vi "升降桅杆.vi"() -> ()   [LabVIEW 2018]
panel:
  in  "停止 2":bool
  in  "抱紧 2":bool
  in  "打开 2":bool
  in  "停止":bool
  in  "抱紧":bool
  in  "打开":bool
  out "推进模块故障 2":bool caption="地位正常运行"
  out "推进模块正常 2":bool
  in  "停止":bool
  in  "选项卡控件 8":T1(tab)
  out "回转故障信息":string
  in  "停止 3":bool
  in  "原始位":bool
  in  "工作位":bool
  out "到达工作位":bool
  out "电机运行状态 4":bool
  out "未到位 4":bool
  out "到达原始位":bool
  out "回转模块故障":bool caption="地位正常运行"
  out "回转模块正常":bool
  out "俯仰位移传感器":i64 caption="Output Value"
  out "挡板推进传感器":i64 caption="Output Value"
  out "升降桅杆位移传感器":i64 caption="Output Value"
  out "推进模块故障信息":string
  out "电机运行状态 3":bool
  out "未到位 3":bool
  out "缩回到位":bool
  out "推进到位":bool
  out "Output Value 18":dbl caption="Output Value" format="%.2f"
  out "Output Value 17":dbl caption="Output Value" format="%.2f"
  out "Output Value 16":dbl caption="Output Value" format="%.2f"
  out "Output Value 15":dbl caption="Output Value" format="%.2f"
  out "Output Value 14":dbl caption="Output Value" format="%.2f"
  out "Output Value 13":dbl caption="Output Value" format="%.2f"
  out "Output Value 12":dbl caption="Output Value" format="%.2f"
  out "Output Value 11":dbl caption="Output Value" format="%.2f"
  out "Output Value 10":dbl caption="Output Value" format="%.2f"
  out "Output Value 9":dbl caption="Output Value" format="%.2f"
  out "Output Value 8":dbl caption="Output Value" format="%.2f"
  out "Output Value 7":dbl caption="Output Value" format="%.2f"
  out "Output Value 6":dbl caption="Output Value" format="%.2f"
  out "Output Value 5":dbl caption="Output Value" format="%.2f"
  out "Output Value 4":dbl caption="Output Value" format="%.2f"
  out "Output Value 3":dbl caption="Output Value" format="%.2f"
  out "Output Value 2":dbl caption="Output Value" format="%.2f"
  out "Output Value":dbl format="%.2f"
  out "系统通讯故障":bool
  out "系统通讯正常":bool
  in  "灯56":bool
  in  "灯34":bool
  in  "灯12":bool
  out "电机运行状态 2":bool
  out "未到位 2":bool
  out "抱爪抱紧到位 2":bool
  out "抱爪打开到位 2":bool
  out "电机运行状态":bool
  out "未到位":bool
  out "抱爪抱紧到位":bool
  out "抱爪打开到位":bool
  out "电机或驱动器故障 2":bool
  out "电机或驱动器正常 2":bool
  out "电机或驱动器故障":bool
  out "电机或驱动器正常":bool
  out "挡板后退到位":bool
  out "挡板推进到位":bool
  out "俯仰缸回降到位":bool
  out "俯仰缸升起到位":bool
  out "桅杆位置4到位":bool
  out "桅杆位置3到位":bool
  out "桅杆位置2到位":bool
  out "桅杆位置1到位":bool
  in  "挡板后退":bool
  in  "挡板推进":bool
  in  "俯仰缸回降":bool
  in  "俯仰缸升起":bool
  in  "桅杆位置":bool
  in  "桅杆位置3":bool
  in  "桅杆位置2":bool
  in  "桅杆位置1":bool
  in  "Application filename":string="canceshi1"
  in  "IP Port":string="22222"
  in  "IP Address":string="192.168.0.10"
  out "旋转":dbl caption="Output Value" format="%.2f"
  out "升降":dbl caption="Output Value" format="%.2f"
  out "抱爪1":dbl caption="Output Value" format="%.2f"
  out "伺服阀":dbl caption="Output Value" format="%.2f"
  out "startapp":i32 caption="port copy"
  out "loadapp":i32 caption="port copy"
  out "tcpip":i32 caption="Port"
  # "推进控制模块"
  # "回转控制模块"
  # "捕获臂控制模块"
  # "单位/mm"
  # "单位/mm"
  # "单位/mm"
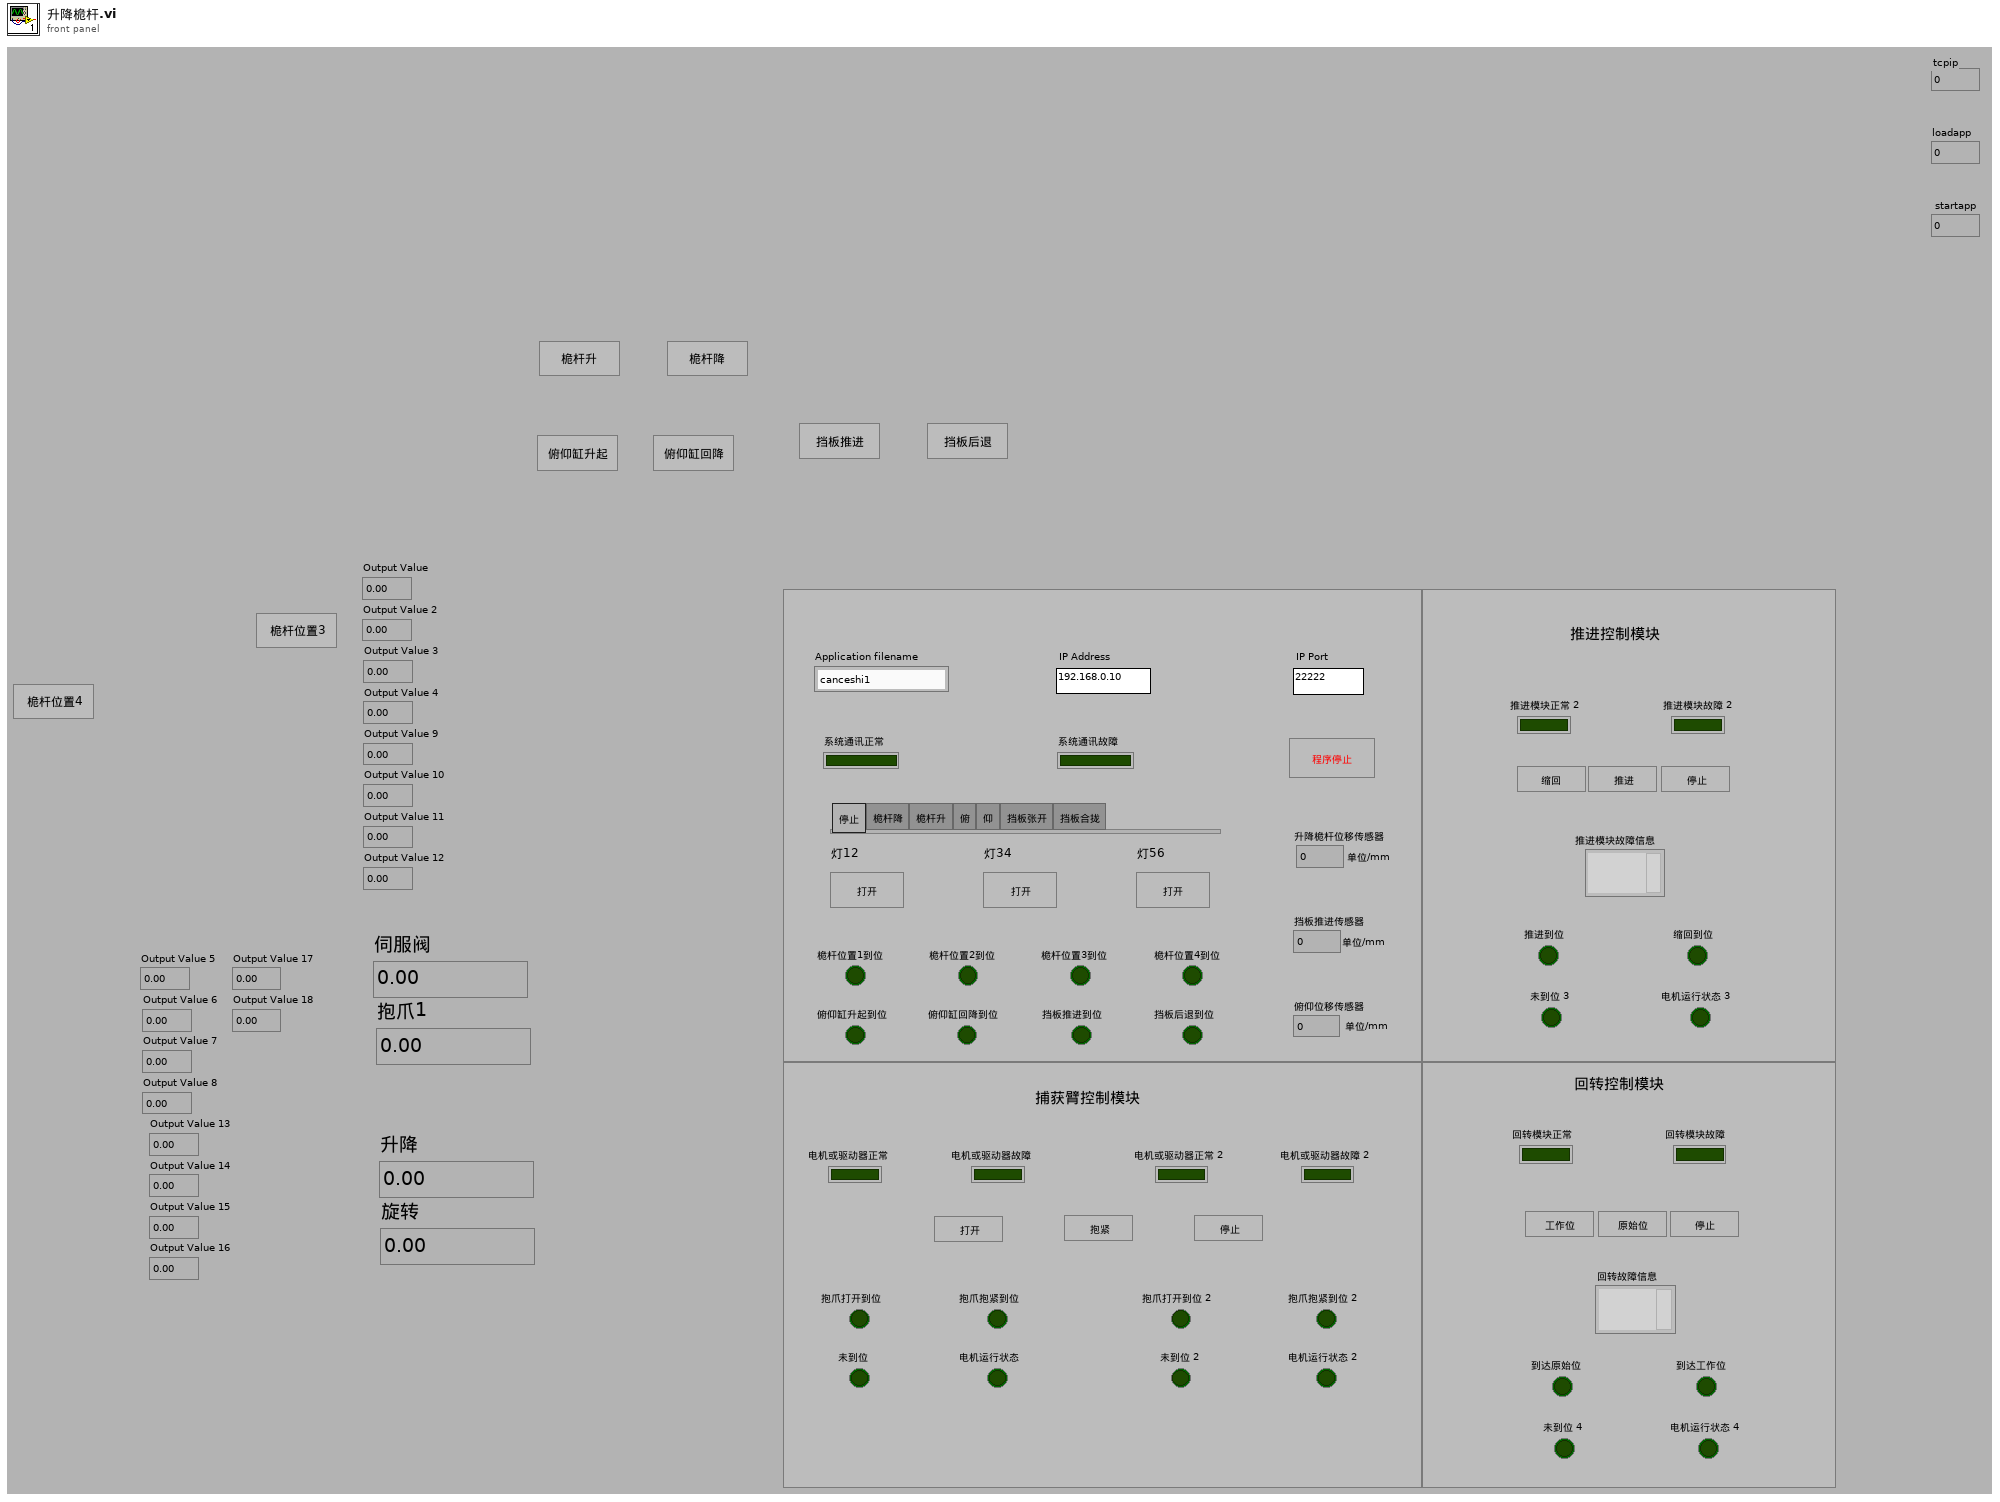
[diagram p1: front panel]
types:
  T1 = enum32{"停止", "桅杆降", "桅杆升", "俯", "仰", "挡板张开", "挡板合拢"}
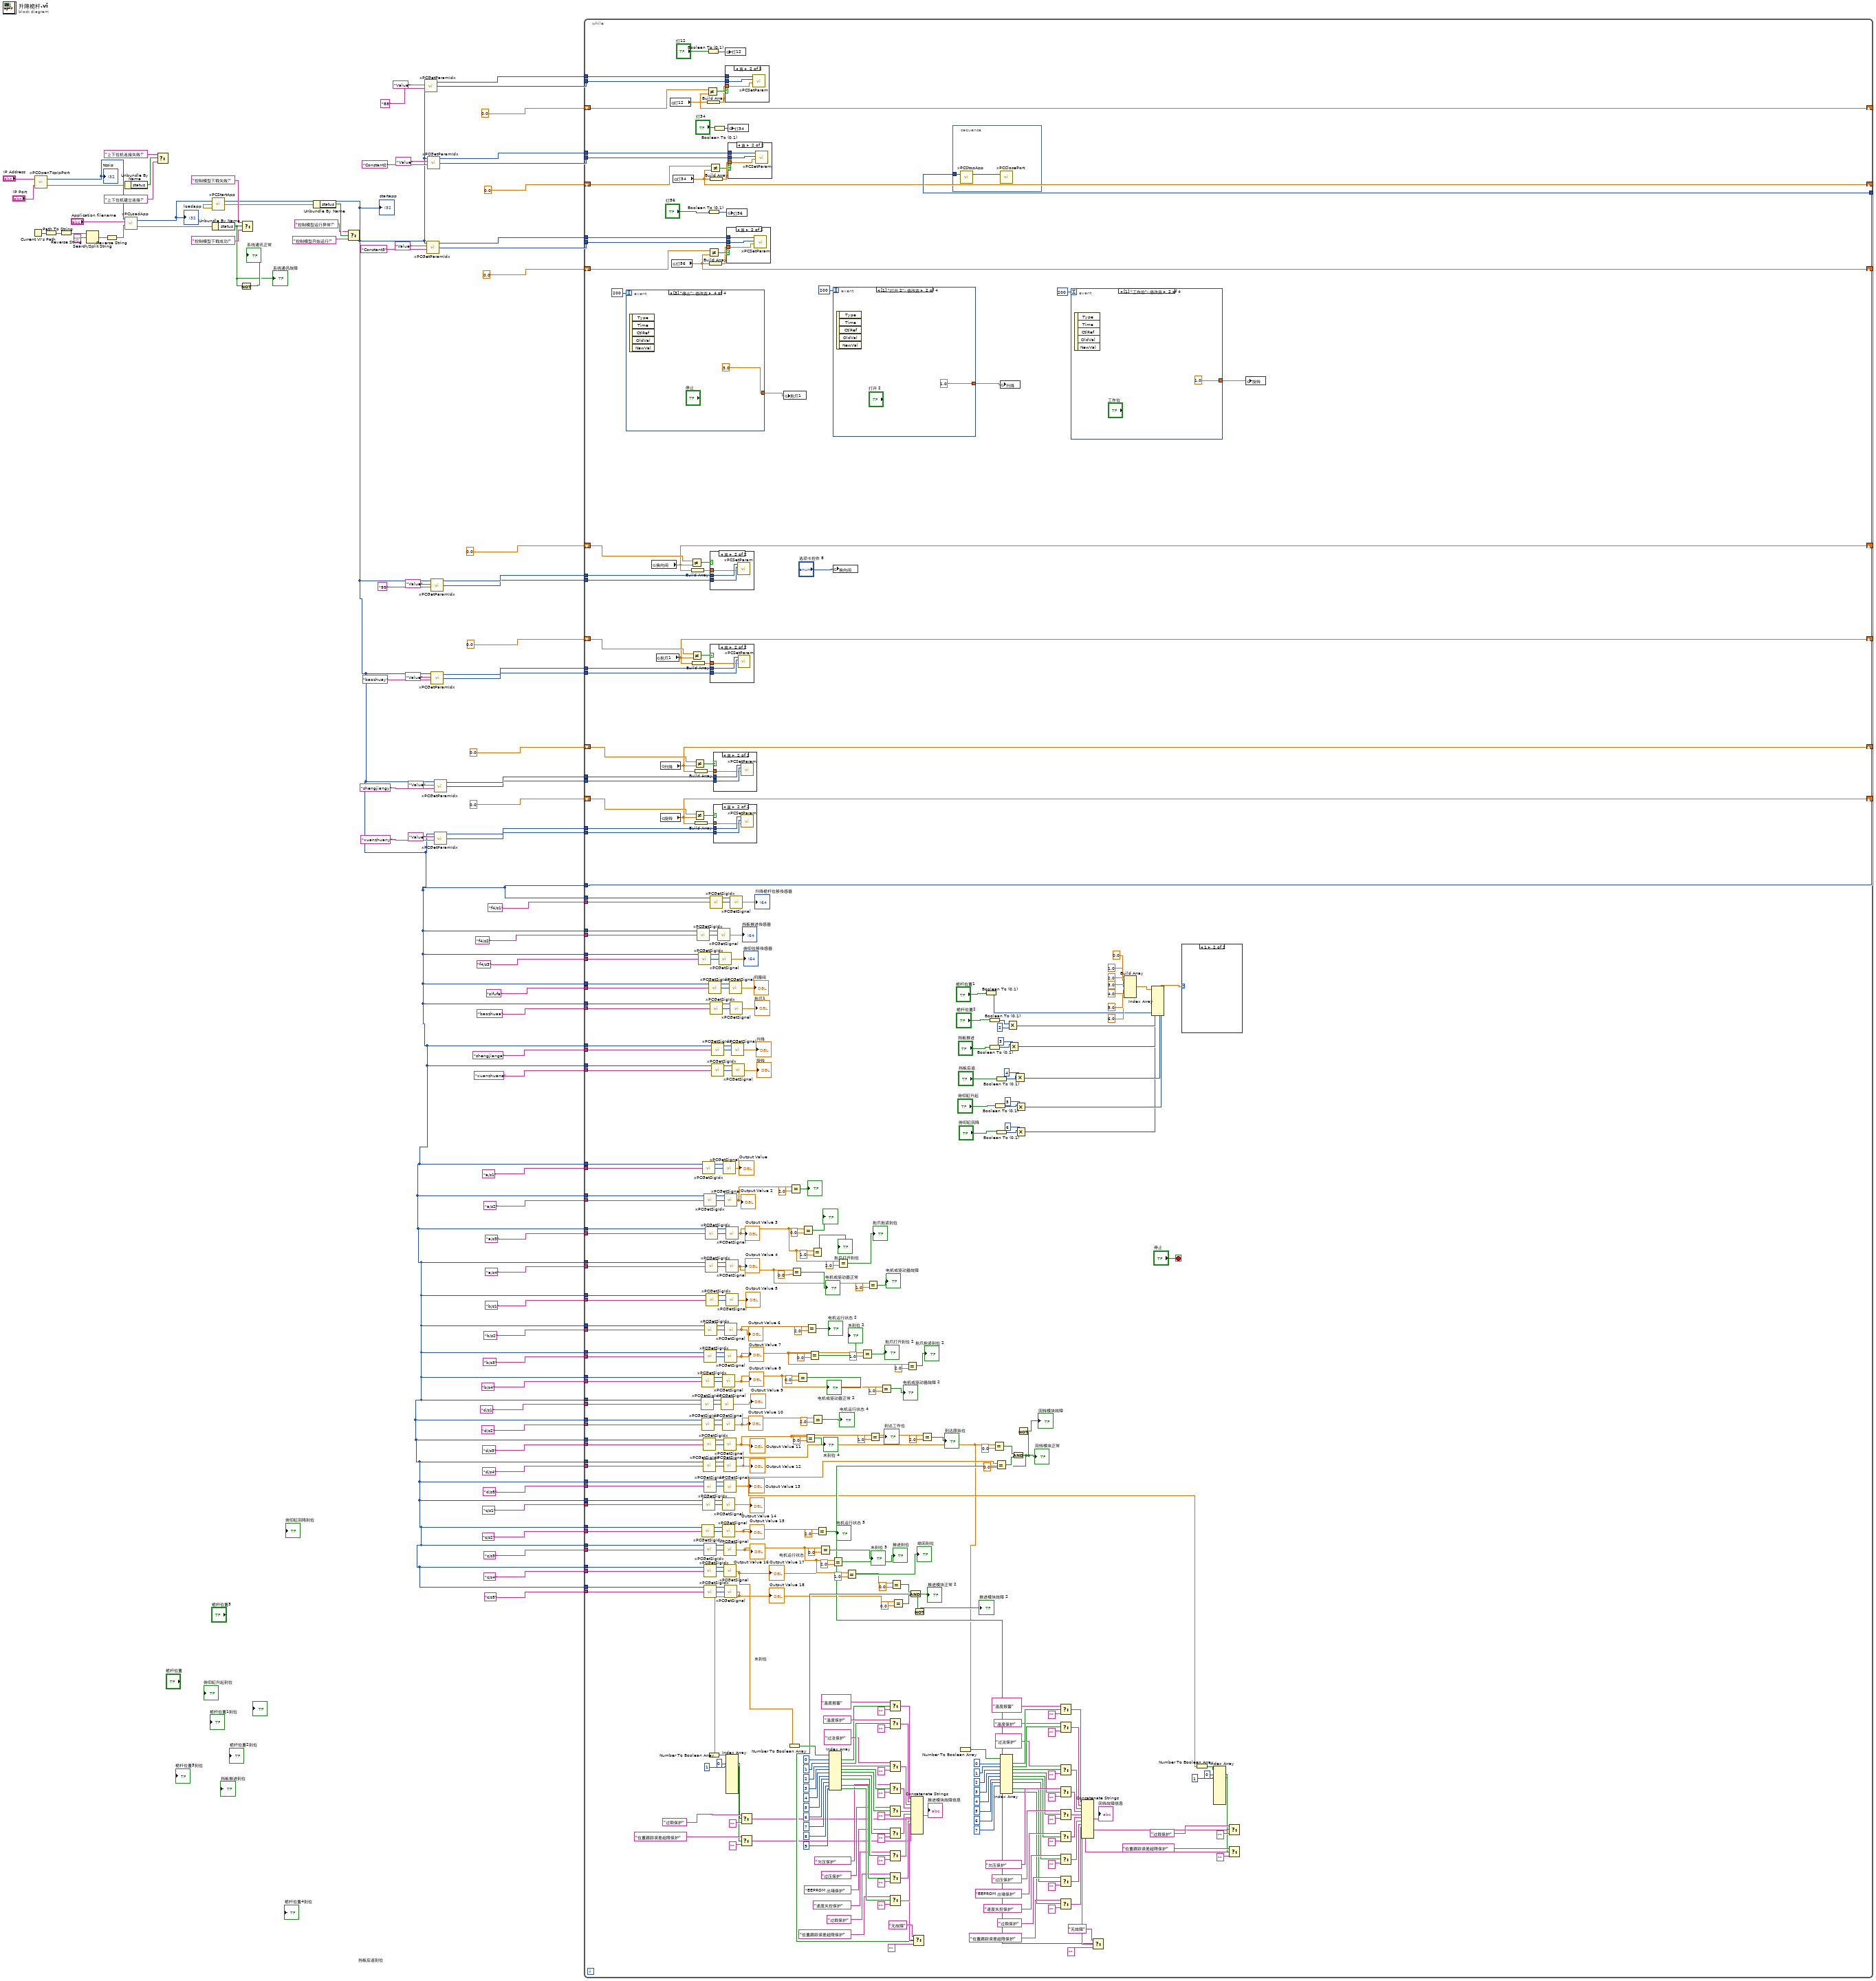
[diagram p0: block diagram]
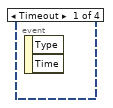
[diagram p2: hidden frame]
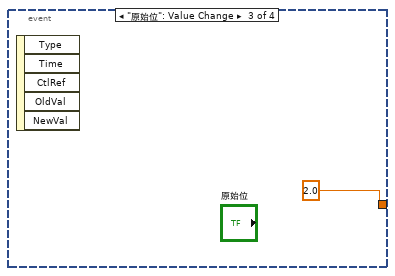
[diagram p3: hidden frame]
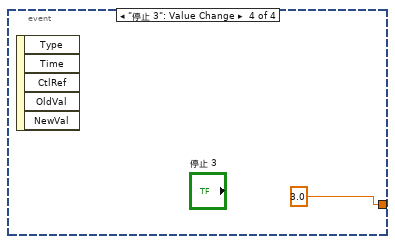
[diagram p4: hidden frame]
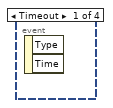
[diagram p5: hidden frame]
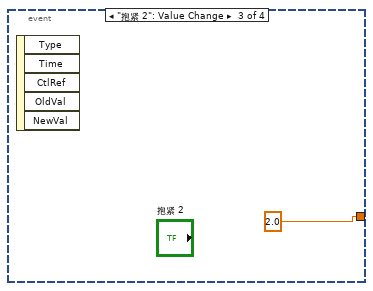
[diagram p6: hidden frame]
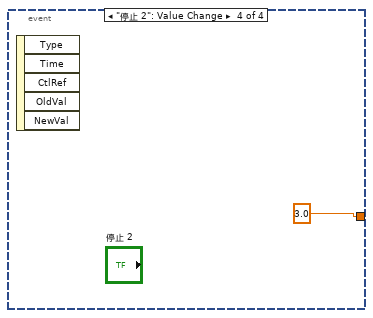
[diagram p7: hidden frame]
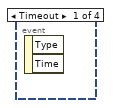
[diagram p8: hidden frame]
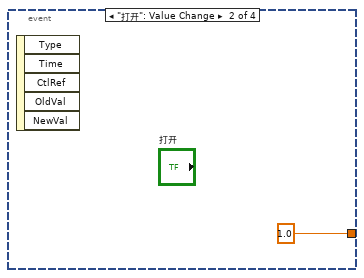
[diagram p9: hidden frame]
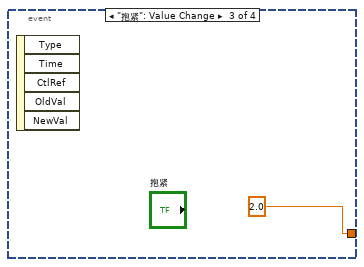
[diagram p10: hidden frame]
diagram:
  n1 = Current VI's Path() -> (path=w80:path)
  n2 = call "xPCOpenTcpIpPort.vi"("port"="IP Port", "address"="IP Address") -> ("error out"=w70:errorcluster, "Port"=w71:i32)
  "tcpip" <- w71
  n3 = Path To String(path=w80) -> (string=w82:string)
  n4 = Reverse String(1:w82) -> (0:w84:string)
  n5 = Search/Split String(string=w84, search string/char (-)="\\" ("search char (-)")) -> (match + rest of string=w83:string)  [unwired: 1 in, 2 out]
  n6 = Reverse String(1:w83) -> (0:w85:string)
  n7 = Unbundle By Name(w70) -> ("status"=w77:bool)
  n8 = call "xPCLoadApp.vi"("pathstr"=w85, "filename"="Application filename", "port"=w71) -> ("error out"=w72:errorcluster, "port copy"=w79:i32)  [unwired: 1 in]
  "loadapp" <- w79
  n9 = Select(t="上下位机连接失败!" ("message"), s=w77, f="上下位机建立连接!" ("message")) -> ()  [unwired: 1 out]
  n10 = call "xPCStartApp.vi"("port"=w79) -> ("error out"=w64:errorcluster, "port copy"=w1:i32)  [unwired: 1 in]
  "startapp" <- w1
  n11 = Unbundle By Name(w72) -> ("status"=w37:bool)
  "系统通讯故障" <- w37
  n12 = Not(x=w37) -> (.not. x?=→"系统通讯正常":bool)
  n13 = Select(t="控制模型下载失败!" ("message"), s=w37, f="控制模型下载成功!" ("message")) -> ()  [unwired: 1 out]
  n14 = Unbundle By Name(w64) -> ("status"=w66:bool)
  n15 = Select(t="控制模型运行异常!" ("message"), s=w66, f="控制模型开始运行!" ("message")) -> ()  [unwired: 1 out]
  n16 = call "xPCGetParamIdx.vi"("blockpath"="88" ("pathstr"), "parametername"="Value" ("filename"), "port"=w1) -> ("identifier"=w57:i32, "port copy"=w58:i32)  [unwired: 1 in, 1 out]
  n17 = call "xPCGetParamIdx.vi"("blockpath"="Constant3" ("pathstr"), "parametername"="Value" ("filename"), "port"=w1) -> ("identifier"=w46:i32, "port copy"=w47:i32)  [unwired: 1 in, 1 out]
  n18 = call "xPCGetParamIdx.vi"("blockpath"="Constant2" ("pathstr"), "parametername"="Value" ("filename"), "port"=w1) -> ("identifier"=w51:i32, "port copy"=w50:i32)  [unwired: 1 in, 1 out]
  n19 = call "xPCGetParamIdx.vi"("blockpath"="99" ("pathstr"), "parametername"="Value" ("filename"), "port"=w1) -> ("identifier"=w43:i32, "port copy"=w61:i32)  [unwired: 1 in, 1 out]
  n20 = call "xPCGetParamIdx.vi"("blockpath"="baozhuay" ("pathstr"), "parametername"="Value" ("filename"), "port"=w1) -> ("identifier"=w16:i32, "port copy"=w14:i32)  [unwired: 1 in, 1 out]
  n21 = call "xPCGetParamIdx.vi"("blockpath"="shengjiangy" ("pathstr"), "parametername"="Value" ("filename"), "port"=w1) -> ("identifier"=w7:i32, "port copy"=w9:i32)  [unwired: 1 in, 1 out]
  n22 = call "xPCGetParamIdx.vi"("blockpath"="xuanzhuany" ("pathstr"), "parametername"="Value" ("filename"), "port"=w1) -> ("identifier"=w6:i32, "port copy"=w4:i32)  [unwired: 1 in, 1 out]
  n23 = while {
    tunnel: w1 -> [w473]
    tunnel: [w473] -> w78
    shift-right: [w467] -> _
    shift-left: 0.0 -> [w470]
    tunnel: w43 -> [w469]
    tunnel: w61 -> [w468]
    shift-right: [w466] -> _
    shift-left: 0.0 -> [w465]
    tunnel: w57 -> [w462]
    tunnel: w58 -> [w461]
    tunnel: w1 -> [w458]
    tunnel: "f4/s1" ("pathstr") -> [w455]
    shift-right: [w448] -> _
    shift-left: 0.0 -> [w449]
    tunnel: w51 -> [w452]
    tunnel: w50 -> [w453]
    shift-right: [w447] -> _
    shift-left: 0.0 -> [w446]
    tunnel: w46 -> [w443]
    tunnel: w47 -> [w442]
    tunnel: w1 -> [w433]
    tunnel: "sifufa" ("pathstr") -> [w436]
    tunnel: w1 -> [w432]
    tunnel: "baozhuaa" ("pathstr") -> [w429]
    tunnel: w1 -> [w427]
    tunnel: "shengjianga" ("pathstr") -> [w424]
    tunnel: w1 -> [w418]
    tunnel: "xuanzhuana" ("pathstr") -> [w421]
    tunnel: w1 -> [w393]
    tunnel: "a/s1" ("pathstr") -> [w391]
    tunnel: w1 -> [w394]
    tunnel: "a/s2" ("pathstr") -> [w396]
    tunnel: w1 -> [w401]
    tunnel: "a/s3" ("pathstr") -> [w399]
    tunnel: w1 -> [w402]
    tunnel: "a/s4" ("pathstr") -> [w404]
    tunnel: w1 -> [w409]
    tunnel: "b/s1" ("pathstr") -> [w407]
    tunnel: w1 -> [w410]
    tunnel: "b/s2" ("pathstr") -> [w412]
    tunnel: w1 -> [w417]
    tunnel: "b/s3" ("pathstr") -> [w415]
    tunnel: w1 -> [w389]
    tunnel: "b/s4" ("pathstr") -> [w387]
    tunnel: w1 -> [w382]
    tunnel: "d/s1" ("pathstr") -> [w384]
    tunnel: w1 -> [w381]
    tunnel: "d/s2" ("pathstr") -> [w379]
    tunnel: w1 -> [w374]
    tunnel: "d/s3" ("pathstr") -> [w376]
    tunnel: w1 -> [w373]
    tunnel: "d/s4" ("pathstr") -> [w371]
    tunnel: w1 -> [w366]
    tunnel: "d/s5" ("pathstr") -> [w368]
    tunnel: w1 -> [w365]
    tunnel: "c/s1" ("pathstr") -> [w363]
    tunnel: w1 -> [w358]
    tunnel: "c/s2" ("pathstr") -> [w360]
    tunnel: w1 -> [w349]
    tunnel: "c/s3" ("pathstr") -> [w347]
    tunnel: w1 -> [w350]
    tunnel: "c/s4" ("pathstr") -> [w352]
    tunnel: w1 -> [w357]
    tunnel: "c/s5" ("pathstr") -> [w355]
    tunnel: w1 -> [w187]
    tunnel: "f4/s2" ("pathstr") -> [w190]
    tunnel: w1 -> [w186]
    tunnel: "f4/s3" ("pathstr") -> [w183]
    shift-right: [w95] -> _
    shift-left: 0.0 -> [w108]
    tunnel: w16 -> [w109]
    tunnel: w14 -> [w110]
    shift-right: [w94] -> _
    shift-left: 0.0 -> [w103]
    tunnel: w7 -> [w102]
    tunnel: w9 -> [w101]
    shift-right: [w93] -> _
    shift-left: 0.0 -> [w98]
    tunnel: w6 -> [w99]
    tunnel: w4 -> [w100]
    stop <- "停止" stop-if-true
    n24 = event shown="[3] \"停止\": 值改变" {
      selector: _ -> [_ _ _ _]
      dyn-events: _ -> [_ _ _ _]
      timeout: 200 -> [_ _ _ _]
      tunnel: [_ 1.0 ("抱爪1") 2.0 ("抱爪1") 3.0 ("抱爪1")] -> w91
      event Timeout {
        n25 = event-data() -> ()  [unwired: 1 in, 2 out]
      }
      event "打开": Value Change {
        n26 = event-data() -> ()  [unwired: 1 in, 5 out]
      }
      event "抱紧": Value Change {
        n27 = event-data() -> ()  [unwired: 1 in, 5 out]
      }
      event "停止": Value Change {
        n28 = event-data() -> ()  [unwired: 1 in, 5 out]
      }
    }
    n29 = global read "全局 1.vi" "换向阀"() -> (w467:dbl)
    n30 = global read "全局 1.vi" "抱爪1"() -> (w95:dbl)
    n31 = global read "全局 1.vi" "升降"() -> (w94:dbl)
    n32 = global read "全局 1.vi" "旋转"() -> (w93:dbl)
    n33 = global read "全局 1.vi" "灯12"() -> (w466:dbl)
    n34 = global read "全局 1.vi" "灯56"() -> (w447:dbl)
    n35 = global read "全局 1.vi" "灯34"() -> (w448:dbl)
    n36 = Not Equal?(x=w470, y=w467) -> (x != y?=w471:bool)
    n37 = Not Equal?(x=w108, y=w95) -> (x != y?=w107:bool)
    n38 = Build Array(w467) -> (w472:dbl[])
    n39 = Build Array(w95) -> (w106:dbl[])
    n40 = Not Equal?(x=w103, y=w94) -> (x != y?=w104:bool)
    n41 = Not Equal?(x=w98, y=w93) -> (x != y?=w97:bool)
    n42 = Build Array(w94) -> (w105:dbl[])
    n43 = Build Array(w93) -> (w96:dbl[])
    n44 = call "xPCGetSigIdx.vi"("blockpath"=w190, "port"=w187) -> ("identifier"=w191:i32, "port copy"=w188:i32)  [unwired: 1 in, 1 out]
    n45 = call "xPCGetSigIdx.vi"("blockpath"=w183, "port"=w186) -> ("identifier"=w182:i32, "port copy"=w185:i32)  [unwired: 1 in, 1 out]
    n46 = call "xPCGetSigIdx.vi"("blockpath"=w384, "port"=w382) -> ("identifier"=w385:i32, "port copy"=w383:i32)  [unwired: 1 in, 1 out]
    n47 = call "xPCGetSigIdx.vi"("blockpath"=w387, "port"=w389) -> ("identifier"=w386:i32, "port copy"=w388:i32)  [unwired: 1 in, 1 out]
    n48 = call "xPCGetSigIdx.vi"("blockpath"=w379, "port"=w381) -> ("identifier"=w378:i32, "port copy"=w380:i32)  [unwired: 1 in, 1 out]
    n49 = call "xPCGetSigIdx.vi"("blockpath"=w360, "port"=w358) -> ("identifier"=w361:i32, "port copy"=w359:i32)  [unwired: 1 in, 1 out]
    n50 = call "xPCGetSigIdx.vi"("blockpath"=w363, "port"=w365) -> ("identifier"=w362:i32, "port copy"=w364:i32)  [unwired: 1 in, 1 out]
    n51 = call "xPCGetSigIdx.vi"("blockpath"=w391, "port"=w393) -> ("identifier"=w390:i32, "port copy"=w392:i32)  [unwired: 1 in, 1 out]
    n52 = call "xPCGetSigIdx.vi"("blockpath"=w376, "port"=w374) -> ("identifier"=w377:i32, "port copy"=w375:i32)  [unwired: 1 in, 1 out]
    n53 = call "xPCGetSigIdx.vi"("blockpath"=w371, "port"=w373) -> ("identifier"=w370:i32, "port copy"=w372:i32)  [unwired: 1 in, 1 out]
    n54 = call "xPCGetSigIdx.vi"("blockpath"=w368, "port"=w366) -> ("identifier"=w369:i32, "port copy"=w367:i32)  [unwired: 1 in, 1 out]
    n55 = call "xPCGetSigIdx.vi"("blockpath"=w347, "port"=w349) -> ("identifier"=w346:i32, "port copy"=w348:i32)  [unwired: 1 in, 1 out]
    n56 = call "xPCGetSigIdx.vi"("blockpath"=w352, "port"=w350) -> ("identifier"=w353:i32, "port copy"=w351:i32)  [unwired: 1 in, 1 out]
    n57 = call "xPCGetSigIdx.vi"("blockpath"=w396, "port"=w394) -> ("identifier"=w397:i32, "port copy"=w395:i32)  [unwired: 1 in, 1 out]
    n58 = call "xPCGetSigIdx.vi"("blockpath"=w415, "port"=w417) -> ("identifier"=w414:i32, "port copy"=w416:i32)  [unwired: 1 in, 1 out]
    n59 = call "xPCGetSigIdx.vi"("blockpath"=w355, "port"=w357) -> ("identifier"=w354:i32, "port copy"=w356:i32)  [unwired: 1 in, 1 out]
    n60 = call "xPCGetSigIdx.vi"("blockpath"=w412, "port"=w410) -> ("identifier"=w413:i32, "port copy"=w411:i32)  [unwired: 1 in, 1 out]
    n61 = call "xPCGetSigIdx.vi"("blockpath"=w399, "port"=w401) -> ("identifier"=w398:i32, "port copy"=w400:i32)  [unwired: 1 in, 1 out]
    n62 = call "xPCGetSigIdx.vi"("blockpath"=w404, "port"=w402) -> ("identifier"=w405:i32, "port copy"=w403:i32)  [unwired: 1 in, 1 out]
    n63 = call "xPCGetSigIdx.vi"("blockpath"=w407, "port"=w409) -> ("identifier"=w406:i32, "port copy"=w408:i32)  [unwired: 1 in, 1 out]
    n64 = Not Equal?(x=w465, y=w466) -> (x != y?=w464:bool)
    n65 = Boolean To (0,1)(Boolean="灯12") -> (0, 1=w459:i16)
    n66 = Build Array(w466) -> (w463:dbl[])
    n67 = Boolean To (0,1)(Boolean="灯56") -> (0, 1=w439:i16)
    n68 = Not Equal?(x=w446, y=w447) -> (x != y?=w445:bool)
    n69 = call "xPCGetSigIdx.vi"("blockpath"=w436, "port"=w433) -> ("identifier"=w437:i32, "port copy"=w434:i32)  [unwired: 1 in, 1 out]
    n70 = Not Equal?(x=w449, y=w448) -> (x != y?=w450:bool)
    n71 = Build Array(w447) -> (w444:dbl[])
    n72 = case shown="真" w471 {
      tunnel: w468 -> [_ w503]
      tunnel: w469 -> [_ w502]
      tunnel: w472 -> [_ w501]
      frame False {
      }
      frame True {
        n73 = call "xPCSetParam.vi"("value"=w501, "index"=w502, "port"=w503) -> ()  [unwired: 1 in, 2 out]
      }
    }
    n74 = call "xPCGetSigIdx.vi"("blockpath"=w455, "port"=w458) -> ("identifier"=w454:i32, "port copy"=w457:i32)  [unwired: 1 in, 1 out]
    n75 = call "xPCGetSigIdx.vi"("blockpath"=w429, "port"=w432) -> ("identifier"=w428:i32, "port copy"=w431:i32)  [unwired: 1 in, 1 out]
    n76 = Build Array(w448) -> (w451:dbl[])
    n77 = case shown="真" w107 {
      tunnel: w110 -> [_ w491]
      tunnel: w109 -> [_ w490]
      tunnel: w106 -> [_ w489]
      frame False {
      }
      frame True {
        n78 = call "xPCSetParam.vi"("value"=w489, "index"=w490, "port"=w491) -> ()  [unwired: 1 in, 2 out]
      }
    }
    n79 = call "xPCGetSigIdx.vi"("blockpath"=w424, "port"=w427) -> ("identifier"=w423:i32, "port copy"=w426:i32)  [unwired: 1 in, 1 out]
    n80 = call "xPCGetSigIdx.vi"("blockpath"=w421, "port"=w418) -> ("identifier"=w422:i32, "port copy"=w419:i32)  [unwired: 1 in, 1 out]
    n81 = case shown="真" w104 {
      tunnel: w101 -> [_ w488]
      tunnel: w102 -> [_ w487]
      tunnel: w105 -> [_ w486]
      frame False {
      }
      frame True {
        n82 = call "xPCSetParam.vi"("value"=w486, "index"=w487, "port"=w488) -> ()  [unwired: 1 in, 2 out]
      }
    }
    n83 = case shown="真" w97 {
      tunnel: w100 -> [_ w485]
      tunnel: w99 -> [_ w484]
      tunnel: w96 -> [_ w483]
      frame False {
      }
      frame True {
        n84 = call "xPCSetParam.vi"("value"=w483, "index"=w484, "port"=w485) -> ()  [unwired: 1 in, 2 out]
      }
    }
    n85 = Boolean To (0,1)(Boolean="灯34") -> (0, 1=w441:i16)
    n86 = call "xPCGetSignal.vi"("signal"=w191, "port"=w188) -> ("Output Value"=→"挡板推进传感器":dbl)  [unwired: 1 in, 2 out]
    n87 = call "xPCGetSignal.vi"("signal"=w182, "port"=w185) -> ("Output Value"=→"俯仰位移传感器":dbl)  [unwired: 1 in, 2 out]
    n88 = call "xPCGetSignal.vi"("signal"=w385, "port"=w383) -> ("Output Value"=→"Output Value 9":dbl)  [unwired: 1 in, 2 out]
    n89 = call "xPCGetSignal.vi"("signal"=w386, "port"=w388) -> ("Output Value"=w313:dbl)  [unwired: 1 in, 2 out]
    "Output Value 8" <- w313
    n90 = call "xPCGetSignal.vi"("signal"=w378, "port"=w380) -> ("Output Value"=w310:dbl)  [unwired: 1 in, 2 out]
    "Output Value 10" <- w310
    n91 = call "xPCGetSignal.vi"("signal"=w361, "port"=w359) -> ("Output Value"=w299:dbl)  [unwired: 1 in, 2 out]
    "Output Value 15" <- w299
    n92 = call "xPCGetSignal.vi"("signal"=w362, "port"=w364) -> ("Output Value"=→"Output Value 14":dbl)  [unwired: 1 in, 2 out]
    n93 = call "xPCGetSignal.vi"("signal"=w390, "port"=w392) -> ("Output Value"=→"Output Value":dbl)  [unwired: 1 in, 2 out]
    n94 = call "xPCGetSignal.vi"("signal"=w377, "port"=w375) -> ("Output Value"=w302:dbl)  [unwired: 1 in, 2 out]
    "Output Value 11" <- w302
    n95 = call "xPCGetSignal.vi"("signal"=w370, "port"=w372) -> ("Output Value"=w111:dbl)  [unwired: 1 in, 2 out]
    "Output Value 12" <- w111
    n96 = call "xPCGetSignal.vi"("signal"=w369, "port"=w367) -> ("Output Value"=w116:dbl)  [unwired: 1 in, 2 out]
    "Output Value 13" <- w116
    n97 = call "xPCGetSignal.vi"("signal"=w346, "port"=w348) -> ("Output Value"=w292:dbl)  [unwired: 1 in, 2 out]
    "Output Value 16" <- w292
    n98 = call "xPCGetSignal.vi"("signal"=w353, "port"=w351) -> ("Output Value"=w129:dbl)  [unwired: 1 in, 2 out]
    "Output Value 17" <- w129
    n99 = call "xPCGetSignal.vi"("signal"=w397, "port"=w395) -> ("Output Value"=w340:dbl)  [unwired: 1 in, 2 out]
    "Output Value 2" <- w340
    n100 = call "xPCGetSignal.vi"("signal"=w414, "port"=w416) -> ("Output Value"=w315:dbl)  [unwired: 1 in, 2 out]
    "Output Value 7" <- w315
    n101 = call "xPCGetSignal.vi"("signal"=w354, "port"=w356) -> ("Output Value"=w128:dbl)  [unwired: 1 in, 2 out]
    "Output Value 18" <- w128
    n102 = Number To Boolean Array(number=w128) -> (Boolean array=w130:bool[])
    n103 = call "xPCGetSignal.vi"("signal"=w413, "port"=w411) -> ("Output Value"=w322:dbl)  [unwired: 1 in, 2 out]
    "Output Value 6" <- w322
    n104 = global write "全局 1.vi" "灯12"(w459) -> ()
    n105 = case shown="真" w464 {
      tunnel: w463 -> [_ w500]
      tunnel: w462 -> [_ w499]
      tunnel: w461 -> [_ w498]
      frame False {
      }
      frame True {
        n106 = call "xPCSetParam.vi"("value"=w500, "index"=w499, "port"=w498) -> ()  [unwired: 1 in, 2 out]
      }
    }
    n107 = call "xPCGetSignal.vi"("signal"=w398, "port"=w400) -> ("Output Value"=w334:dbl)  [unwired: 1 in, 2 out]
    "Output Value 3" <- w334
    n108 = call "xPCGetSignal.vi"("signal"=w405, "port"=w403) -> ("Output Value"=w324:dbl)  [unwired: 1 in, 2 out]
    "Output Value 4" <- w324
    n109 = Index Array(array=w130, index #1=0 ("索引"), index #2=1 ("索引")) -> (element #1=w127:bool, element #2=w126:bool)  [unwired: 8 in, 8 out]
    n110 = call "xPCGetSignal.vi"("signal"=w406, "port"=w408) -> ("Output Value"=→"Output Value 5":dbl)  [unwired: 1 in, 2 out]
    n111 = global write "全局 1.vi" "灯56"(w439) -> ()
    n112 = case shown="真" w445 {
      tunnel: w444 -> [_ w494]
      tunnel: w443 -> [_ w493]
      tunnel: w442 -> [_ w492]
      frame False {
      }
      frame True {
        n113 = call "xPCSetParam.vi"("value"=w494, "index"=w493, "port"=w492) -> ()  [unwired: 1 in, 2 out]
      }
    }
    n114 = global write "全局 1.vi" "灯34"(w441) -> ()
    n115 = case shown="真" w450 {
      tunnel: w451 -> [_ w497]
      tunnel: w452 -> [_ w496]
      tunnel: w453 -> [_ w495]
      frame False {
      }
      frame True {
        n116 = call "xPCSetParam.vi"("value"=w497, "index"=w496, "port"=w495) -> ()  [unwired: 1 in, 2 out]
      }
    }
    n117 = call "xPCGetSignal.vi"("signal"=w437, "port"=w434) -> ("Output Value"=→"伺服阀":dbl)  [unwired: 1 in, 2 out]
    n118 = call "xPCGetSignal.vi"("signal"=w454, "port"=w457) -> ("Output Value"=→"升降桅杆位移传感器":dbl)  [unwired: 1 in, 2 out]
    n119 = call "xPCGetSignal.vi"("signal"=w428, "port"=w431) -> ("Output Value"=→"抱爪1":dbl)  [unwired: 1 in, 2 out]
    n120 = call "xPCGetSignal.vi"("signal"=w423, "port"=w426) -> ("Output Value"=→"升降":dbl)  [unwired: 1 in, 2 out]
    n121 = call "xPCGetSignal.vi"("signal"=w422, "port"=w419) -> ("Output Value"=→"旋转":dbl)  [unwired: 1 in, 2 out]
    n122 = Select(t="过载保护" ("message"), s=w127, f="" ("message")) -> (s? t:f=w125:string)
    n123 = Select(t="位置跟踪误差超限保护" ("message"), s=w126, f="" ("message")) -> (s? t:f=w124:string)
    n124 = global write "全局 1.vi" "抱爪1"(w91) -> ()
    n125 = Number To Boolean Array(number=w129) -> (Boolean array=w249:bool[])
    n126 = Equal?(x=w340, y=2.0) -> (x = y?=→"电机运行状态":bool)
    n127 = Equal?(x=w324, y=0.0) -> (x = y?=→"电机或驱动器正常":bool)
    n128 = Equal?(x=w313, y=0.0) -> (x = y?=→"电机或驱动器正常 2":bool)
    n129 = Equal?(x=w334, y=0.0) -> (x = y?=→"未到位":bool)
    n130 = Equal?(x=w302, y=0.0) -> (x = y?=→"未到位 4":bool)
    n131 = Equal?(x=w322, y=2.0) -> (x = y?=→"电机运行状态 2":bool)
    n132 = Equal?(x=w315, y=0.0) -> (x = y?=→"未到位 2":bool)
    n133 = Equal?(x=w334, y=1.0) -> (x = y?=→"抱爪打开到位":bool)
    n134 = Equal?(x=w310, y=2.0) -> (x = y?=→"电机运行状态 4":bool)
    n135 = Equal?(x=w299, y=2.0) -> (x = y?=→"电机运行状态 3":bool)
    n136 = Equal?(x=w292, y=0.0) -> (x = y?=→"未到位 3":bool)
    n137 = Index Array(array=w249, index #1=0 ("索引"), index #2=1 ("索引"), index #3=2 ("索引"), index #4=3 ("索引"), index #5=4 ("索引"), index #6=5 ("索引"), index #7=6 ("索引"), index #8=7 ("索引"), index #9=8 ("索引"), index #10=9 ("索引")) -> (element #1=w251:bool, element #2=w274:bool, element #3=w257:bool, element #4=w260:bool, element #5=w262:bool, element #6=w270:bool, element #7=w281:bool, element #9=w282:bool, element #10=w283:bool)  [unwired: 1 out]
    n138 = Equal?(x=w292, y=2.0) -> (x = y?=→"推进到位":bool)
    n139 = global write "全局 1.vi" "换向阀"("选项卡控件 8") -> ()
    n140 = event shown="[1] \"打开 2\": 值改变" {
      selector: _ -> [_ _ _ _]
      dyn-events: _ -> [_ _ _ _]
      timeout: 200 -> [_ _ _ _]
      tunnel: [_ 1.0 ("抱爪1") 2.0 ("抱爪1") 3.0 ("抱爪1")] -> w90
      event Timeout {
        n141 = event-data() -> ()  [unwired: 1 in, 2 out]
      }
      event "打开 2": Value Change {
        n142 = event-data() -> ()  [unwired: 1 in, 5 out]
      }
      event "抱紧 2": Value Change {
        n143 = event-data() -> ()  [unwired: 1 in, 5 out]
      }
      event "停止 2": Value Change {
        n144 = event-data() -> ()  [unwired: 1 in, 5 out]
      }
    }
    n145 = Equal?(x=w334, y=2.0) -> (x = y?=→"抱爪抱紧到位":bool)
    n146 = Equal?(x=w292, y=1.0) -> (x = y?=→"缩回到位":bool)
    n147 = Equal?(x=w315, y=1.0) -> (x = y?=→"抱爪打开到位 2":bool)
    n148 = Equal?(x=w324, y=1.0) -> (x = y?=→"电机或驱动器故障":bool)
    n149 = Equal?(x=w302, y=1.0) -> (x = y?=→"到达工作位":bool)
    n150 = Equal?(x=w313, y=1.0) -> (x = y?=→"电机或驱动器故障 2":bool)
    n151 = Select(t="温度报警" ("message"), s=w251, f="" ("message")) -> (s? t:f=w263:string)
    n152 = Select(t="温度保护" ("message"), s=w274, f="" ("message")) -> (s? t:f=w264:string)
    n153 = Select(t="过流保护" ("message"), s=w257, f="" ("message")) -> (s? t:f=w265:string)
    n154 = Select(t="欠压保护" ("message"), s=w260, f="" ("message")) -> (s? t:f=w266:string)
    n155 = Select(t="过压保护" ("message"), s=w262, f="" ("message")) -> (s? t:f=w267:string)
    n156 = Select(t="EEPROM 出错保护" ("message"), s=w270, f="" ("message")) -> (s? t:f=w284:string)
    n157 = Select(t="速度失控保护" ("message"), s=w281, f="" ("message")) -> (s? t:f=w285:string)
    n158 = Select(t="过载保护" ("message"), s=w282, f="" ("message")) -> (s? t:f=w286:string)
    n159 = Select(t="位置跟踪误差超限保护" ("message"), s=w283, f="" ("message")) -> (s? t:f=w287:string)
    n160 = Equal?(x=w129, y=0.0) -> (x = y?=w146:bool)
    n161 = Equal?(x=w128, y=0.0) -> (x = y?=w145:bool)
    n162 = Equal?(x=w315, y=2.0) -> (x = y?=→"抱爪抱紧到位 2":bool)
    n163 = And(x=w146, y=w145) -> (x .and. y?=w138:bool)
    "推进模块正常 2" <- w138
    n164 = Select(t="无故障" ("message"), s=w138, f="" ("message")) -> (s? t:f=w193:string)
    n165 = Concatenate Strings(w263, w264, w265, w266, w267, w284, w285, w286, w287, w193, w125, w124) -> (→"推进模块故障信息":string)
    n166 = Not(x=w138) -> (.not. x?=→"推进模块故障 2":bool)
    n167 = Equal?(x=w302, y=2.0) -> (x = y?=→"到达原始位":bool)
    n168 = Number To Boolean Array(number=w111) -> (Boolean array=w240:bool[])
    n169 = Boolean To (0,1)(Boolean="桅杆位置1") -> (0, 1=w156:i16)
    n170 = Boolean To (0,1)(Boolean="桅杆位置2") -> (0, 1=w166:i16)
    n171 = Boolean To (0,1)(Boolean="挡板推进") -> (0, 1=w165:i16)
    n172 = Equal?(x=w111, y=0.0) -> (x = y?=w142:bool)
    n173 = Boolean To (0,1)(Boolean="俯仰缸升起") -> (0, 1=w163:i16)
    n174 = Boolean To (0,1)(Boolean="挡板后退") -> (0, 1=w164:i16)
    n175 = Boolean To (0,1)(Boolean="俯仰缸回降") -> (0, 1=w162:i16)
    n176 = Equal?(x=w116, y=0.0) -> (x = y?=w143:bool)
    n177 = global write "全局 1.vi" "升降"(w90) -> ()
    n178 = Index Array(array=w240, index #1=0 ("索引"), index #2=1 ("索引"), index #3=2 ("索引"), index #4=3 ("索引"), index #5=4 ("索引"), index #6=5 ("索引"), index #7=6 ("索引"), index #8=7 ("索引")) -> (element #1=w238:bool, element #2=w215:bool, element #3=w232:bool, element #4=w229:bool, element #5=w227:bool, element #6=w219:bool, element #7=w210:bool, element #9=w209:bool, element #10=w208:bool)  [unwired: 2 in, 1 out]
    n179 = Multiply(x=w166, y=i16 2) -> (x*y=w155:i16)
    n180 = Multiply(x=w165, y=i16 3) -> (x*y=w154:i16)
    n181 = And(x=w142, y=w143) -> (x .and. y?=w137:bool)
    "回转模块正常" <- w137
    n182 = Multiply(x=w164, y=i16 4) -> (x*y=w153:i16)
    n183 = Multiply(x=w163, y=i16 5) -> (x*y=w152:i16)
    n184 = Multiply(x=w162, y=i16 6) -> (x*y=w151:i16)
    n185 = Not(x=w137) -> (.not. x?=→"回转模块故障":bool)
    n186 = Select(t="温度报警" ("message"), s=w238, f="" ("message")) -> (s? t:f=w226:string)
    n187 = Select(t="温度保护" ("message"), s=w215, f="" ("message")) -> (s? t:f=w225:string)
    n188 = Select(t="过流保护" ("message"), s=w232, f="" ("message")) -> (s? t:f=w224:string)
    n189 = Select(t="欠压保护" ("message"), s=w229, f="" ("message")) -> (s? t:f=w223:string)
    n190 = Select(t="过压保护" ("message"), s=w227, f="" ("message")) -> (s? t:f=w222:string)
    n191 = Select(t="EEPROM 出错保护" ("message"), s=w219, f="" ("message")) -> (s? t:f=w207:string)
    n192 = Select(t="速度失控保护" ("message"), s=w210, f="" ("message")) -> (s? t:f=w206:string)
    n193 = Select(t="过载保护" ("message"), s=w209, f="" ("message")) -> (s? t:f=w205:string)
    n194 = Select(t="位置跟踪误差超限保护" ("message"), s=w208, f="" ("message")) -> (s? t:f=w204:string)
    n195 = event shown="[1] \"工作位\": 值改变" {
      selector: _ -> [_ _ _ _]
      dyn-events: _ -> [_ _ _ _]
      timeout: 200 -> [_ _ _ _]
      tunnel: [_ 1.0 ("抱爪1") 2.0 ("抱爪1") 3.0 ("抱爪1")] -> w89
      event Timeout {
        n196 = event-data() -> ()  [unwired: 1 in, 2 out]
      }
      event "工作位": Value Change {
        n197 = event-data() -> ()  [unwired: 1 in, 5 out]
      }
      event "原始位": Value Change {
        n198 = event-data() -> ()  [unwired: 1 in, 5 out]
      }
      event "停止 3": Value Change {
        n199 = event-data() -> ()  [unwired: 1 in, 5 out]
      }
    }
    n200 = Select(t="无故障" ("message"), s=w137, f="" ("message")) -> (s? t:f=w192:string)
    n201 = Build Array(0.0 ("元素"), 1.0 ("元素"), 2.0 ("元素"), 3.0 ("元素"), 4.0 ("元素"), 5.0 ("元素"), 6.0 ("元素")) -> (w181:dbl[])
    n202 = Index Array(array=w181, index #2=w156, index #3=w155, index #4=w154, index #5=w153, index #6=w152, index #7=w151) -> (element #1=w180:dbl)  [unwired: 1 in, 6 out]
    n203 = case shown="1" w180 {
      frame 0, Default {
      }
      frame 1 {
      }
    }
    n204 = Number To Boolean Array(number=w116) -> (Boolean array=w117:bool[])
    n205 = Index Array(array=w117, index #1=0 ("索引"), index #2=1 ("索引")) -> (element #1=w115:bool, element #2=w114:bool)  [unwired: 8 in, 8 out]
    n206 = Select(t="过载保护" ("message"), s=w115, f="" ("message")) -> (s? t:f=w113:string)
    n207 = Select(t="位置跟踪误差超限保护" ("message"), s=w114, f="" ("message")) -> (s? t:f=w112:string)
    n208 = Concatenate Strings(w226, w225, w224, w223, w222, w207, w206, w205, w204, w192, w113, w112) -> (→"回转故障信息":string)
    n209 = global write "全局 1.vi" "旋转"(w89) -> ()
  }
  n210 = stacked-sequence {
    tunnel: w78 -> [w504]
    frame #0 {
      n211 = call "xPCStopApp.vi"("port"=w504) -> ("port copy"=w505:i32)  [unwired: 1 in, 1 out]
      n212 = call "xPCClosePort.vi"("port"=w505) -> ()  [unwired: 1 in, 2 out]
    }
  }
